vi "Listening Wrapper.vi"(8 "error in (no error)":errorcluster, 11 "CIFCorePlugin in":refnum<class "CIFCorePlugin.lvclass">) -> (0 "error out":errorcluster, 3 "CIFCorePlugin out":refnum<class "CIFCorePlugin.lvclass">)   [LabVIEW 2021, in "CIFCorePlugin.lvclass"]
uses:
  CIFCorePlugin.lvclass
  Typedef/Energized States.ctl
  Common/Typedef/Plugin State.ctl
  CIFCorePlugin.lvclass/CIFCorePlugin.ctl
  <vilib>/CIF Foundation/CIF Utilities/Time/System Time/Sleep Until Future Time.vi
  <vilib>/CIF Foundation/CIF Utilities/Time/SubVIs/Add Error.vi
  <vilib>/CIF Foundation/CIF Utilities/Time/System Time/Get System Time.vi
  <vilib>/CIF Foundation/CIF Utilities/Errors/Append Error Location.vi
  Common/CIFCoreCommon.lvlib
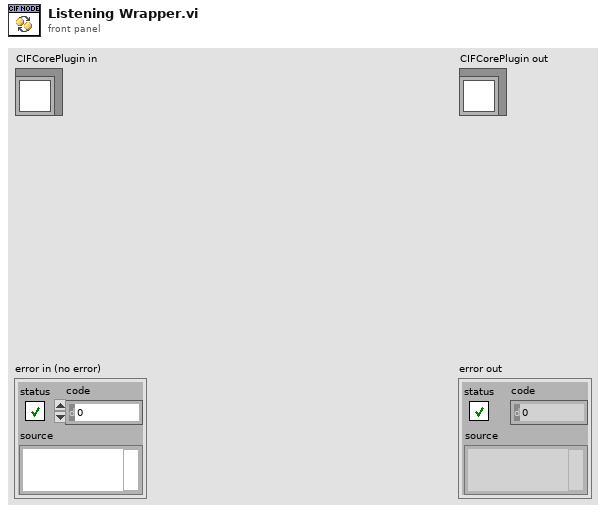
[diagram p1: front panel]
types:
  T1 = typedef "CIFCorePlugin.lvclass/Energized States.ctl" = enum16{"Listen", "Prepare", "Execute", "Housekeep", "Cleanup", "Destroy"}
  T2 = typedef "CIFCoreCommon.lvlib/Plugin State.ctl" = enum32{"Null", "Creating", "Listening", "Running", "CleaningUp", "Destroying", "Prepared", "FTE_Run"}
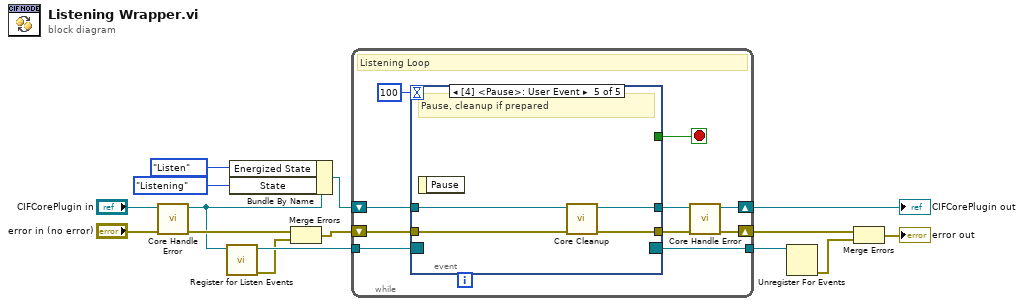
[diagram p0: block diagram]
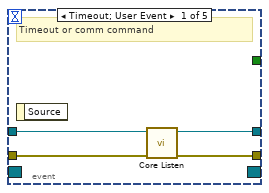
[diagram p2: hidden frame]
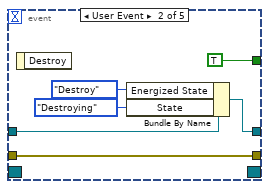
[diagram p3: hidden frame]
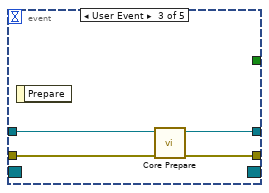
[diagram p4: hidden frame]
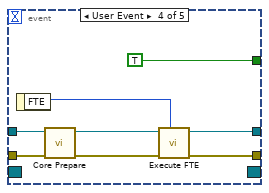
[diagram p5: hidden frame]
diagram:
  n1 = call "Core Handle Error.vi"("error in (no error)"="error in (no error)", "CIFTemplateNode in"="CIFCorePlugin in") -> ("error out"=w7:errorcluster, "CIFTemplateNode out"=w4:refnum<class "CIFCorePlugin.lvclass">)  [unwired: 8 in]
  n2 = call "Register for Listen Events.vi"("CIFCorePlugin in"=w4) -> ("error out"=w6:errorcluster, "Listen Event refnum"=w14:refnum<event-registration>)  [unwired: 9 in]
  n3 = Bundle By Name(cluster=w4, "Energized State"=Energized_States."Listen", "State"=Plugin_State."Listening" ("Main to gRPC Data.Status.State")) -> (w12:refnum<class "CIFCorePlugin.lvclass">)
  n4 = Merge Errors(w7, w6) -> (w5:errorcluster)
  n5 = while {
    shift-right: [w18] -> w13
    shift-left: w12 -> [w25]
    shift-right: [w17] -> w3
    shift-left: w5 -> [w24]
    tunnel: w14 -> [w23]
    tunnel: [w16] -> w15
    stop <- w21 stop-if-true
    # "Listening Loop"
    n6 = event shown="[4] <Pause>: User Event" {
      selector: w23 -> [_ _ _ _ _]
      dyn-events: [_ _ _ _ _] -> w16
      timeout: 100 -> [_ _ _ _ _]
      tunnel: w25 -> [w29 w34 w39 w47 w51]
      tunnel: w24 -> [w28 w35 w38 w46 w50]
      tunnel: [w27 w33 w37 w41 w49] -> w20
      tunnel: [w26 w35 w36 w40 w48] -> w19
      tunnel: [_ TRUE _ TRUE _] -> w21
      event Timeout; User Event {
        # "Timeout or comm command"
        n7 = event-data() -> ()  [unwired: 1 in, 1 out]
        n8 = call "Core Listen.vi"("error in (no error)"=w28, "CIFTemplateNode in"=w29) -> ("error out"=w26:errorcluster, "CIFTemplateNode out"=w27:refnum<class "CIFCorePlugin.lvclass">)  [unwired: 8 in]
      }
      event User Event {
        n9 = event-data() -> ()  [unwired: 1 in, 1 out]
        n10 = Bundle By Name(cluster=w34, "Energized State"=Energized_States."Destroy", "State"=Plugin_State."Destroying" ("Main to gRPC Data.Status.State")) -> (w33:refnum<class "CIFCorePlugin.lvclass">)
      }
      event User Event {
        n11 = event-data() -> ()  [unwired: 1 in, 1 out]
        n12 = call "Core Prepare.vi"("error in (no error)"=w38, "CIFTemplateNode in"=w39) -> ("error out"=w36:errorcluster, "CIFTemplateNode out"=w37:refnum<class "CIFCorePlugin.lvclass">)  [unwired: 8 in]
      }
      event User Event {
        n13 = event-data() -> ("FTE"=w42:i64)  [unwired: 1 in]
        n14 = call "Core Prepare.vi"("error in (no error)"=w46, "CIFTemplateNode in"=w47) -> ("error out"=w43:errorcluster, "CIFTemplateNode out"=w44:refnum<class "CIFCorePlugin.lvclass">)  [unwired: 8 in]
        n15 = call "Execute FTE.vi"("FTE"=w42, "error in (no error)"=w43, "CIFCorePlugin in"=w44) -> ("error out"=w40:errorcluster, "CIFCorePlugin out"=w41:refnum<class "CIFCorePlugin.lvclass">)  [unwired: 7 in]
      }
      event User Event {
        # "Pause, cleanup if prepared"
        n16 = event-data() -> ()  [unwired: 1 in, 1 out]
        n17 = call "Core Cleanup.vi"("error in (no error)"=w50, "CIFTemplateNode in"=w51) -> ("error out"=w48:errorcluster, "CIFTemplateNode out"=w49:refnum<class "CIFCorePlugin.lvclass">)  [unwired: 8 in]
      }
    }
    n18 = call "Core Handle Error.vi"("error in (no error)"=w19, "CIFTemplateNode in"=w20) -> ("error out"=w17:errorcluster, "CIFTemplateNode out"=w18:refnum<class "CIFCorePlugin.lvclass">)  [unwired: 8 in]
  }
  "CIFCorePlugin out" <- w13
  n19 = Unregister For Events(event registration refnum=w15) -> (error out=w2:errorcluster)  [unwired: 1 in]
  n20 = Merge Errors(w3, w2) -> (→"error out":errorcluster)
